vi "Stop Proxy.vi"(8 "error in (no error)":errorcluster, 11 "Sift Client in":refnum<class "Sift Client.lvclass">) -> (0 "error out":errorcluster, 3 "Sift Client out":refnum<class "Sift Client.lvclass">)   [LabVIEW 2024, in "Sift Client.lvlib" / "Sift Client.lvclass"]
doc: "Stops Sift Proxy. This should never nominally be called."
uses:
  Sift Client.lvclass
  Sift Client.lvclass/Sift Client.ctl
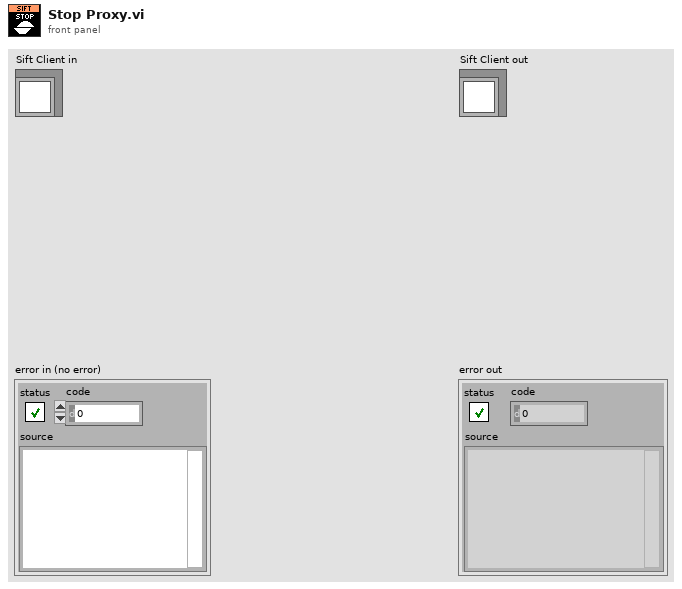
[diagram p1: front panel]
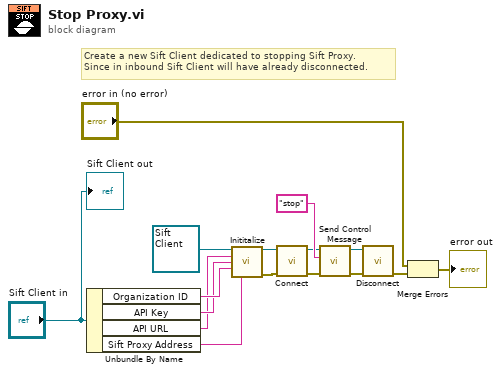
[diagram p0: block diagram]
diagram:
  # "Create a new Sift Client dedicated to stopping Sift Proxy.\nSince in inbound Sift Client will have already disconnected."
  n1 = Unbundle By Name("Sift Client in") -> ("Organization ID"=w14:string, "API Key"=w13:string, "API URL"=w12:string, "Sift Proxy Address"=w11:string)
  n2 = call-dynamic "Inititalize.vi"("Sift Client in"=refnum<class "Sift Client.lvclass"> refnum ("Sift Client.lvlib:Sift Client.lvclass"), "API URL"=w12, "API Key"=w13, "Organization ID"=w14, "Sift Proxy Address"=w11) -> ("Sift Client out"=w7:refnum<class "Sift Client.lvclass">, "error out"=w5:errorcluster)  [unwired: 9 in]
  n3 = call-dynamic "Connect.vi"("error in (no error)"=w5, "Sift Client in"=w7) -> ("error out"=w4:errorcluster, "Sift Client out"=w6:refnum<class "Sift Client.lvclass">)  [unwired: 7 in, 1 out]
  n4 = call-dynamic "Send Control Message.vi"("error in (no error)"=w4, "Command"="stop", "Sift Client in"=w6) -> ("error out"=w2:errorcluster, "Sift Client out"=w3:refnum<class "Sift Client.lvclass">)  [unwired: 7 in]
  n5 = call-dynamic "Disconnect.vi"("error in (no error)"=w2, "Sift Client in"=w3) -> ("error out"=w1:errorcluster)  [unwired: 8 in, 1 out]
  n6 = Merge Errors("error in (no error)", w1) -> (→"error out":errorcluster)
  "Sift Client out" <- "Sift Client in"
